vi "FTW-Endpoint-Connect.vi"(0 "FTW ØMQ Endpoint":refnum<class "FTW-Endpoint-ZMQ.lvclass">, 5 "Endpoint Address":T1, 11 "error in":errorcluster) -> (4 "FTW ØMQ Endpoint out":refnum<class "FTW-Endpoint-ZMQ.lvclass">, 15 "error out":errorcluster)   [LabVIEW 2012, in "FTW-Actor.lvlib" / "FTW-Endpoint-ZMQ.lvclass"]
uses:
  FTW-Endpoint-ZMQ.lvclass
  Utility/FTW-Actor-Address.ctl
  FTW-Endpoint-ZMQ.lvclass/FTW-Endpoint-ZMQ.ctl
  FTW-Actor.lvlib
panel:
  # "Inputs"
  # "Outputs"
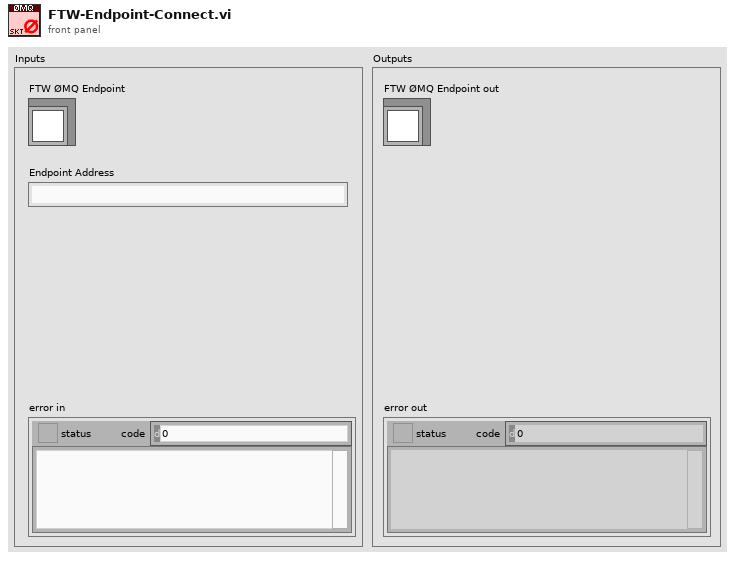
[diagram p1: front panel]
types:
  T1 = typedef "FTW-Actor.lvlib/FTW-Actor-Address.ctl" = string
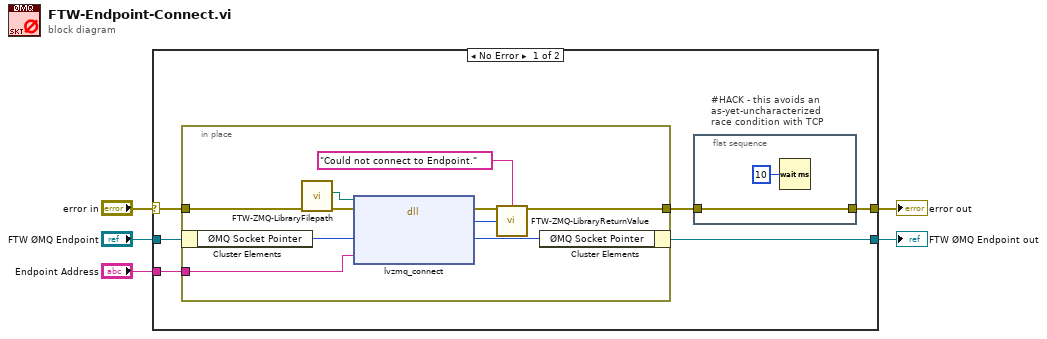
[diagram p0: block diagram]
diagram:
  n1 = case shown="No Error" "error in" {
    selector: "error in" -> [w9 w24]
    tunnel: "FTW ØMQ Endpoint" -> [w11 w25]
    tunnel: [w6 w24] -> w4
    tunnel: [w10 w25] -> w3
    tunnel: "Endpoint Address" -> [w8 _]
    frame No Error {
      n2 = in-place {
        in-place-border: w9 -> [w22]
        in-place-border: [w21] -> w7
        in-place-border: w8 -> [w20]
        n3 = in-place-cluster #1(w11) -> ("ØMQ Socket Pointer"=w23:u64)
        n4 = call "FTW-ZMQ-LibraryFilepath.vi"("error in"=w22) -> ("error out"=w15:errorcluster, "FTW-ZMQ Library Filepath"=w14:path)  [unwired: 8 in, 1 out]
        n5 = dll-call lib="?" fn="lvzmq_connect" ("zmq_labview.dll:lvzmq_bind")(path in=w14, error in=w15, "Socket Pointer"=w23, "Endpoint"=w20) -> (error out=w18:errorcluster, "Return Value"=w17:i32, "Socket Pointer"=w19:u64)  [unwired: 2 in, 1 out]
        n6 = call "FTW-ZMQ-LibraryReturnValue.vi"("error in"=w18, "Error Message"="Could not connect to Endpoint.", "Return Value"=w17) -> ("error out"=w21:errorcluster)  [unwired: 12 in]
        n7 = in-place-cluster #1("ØMQ Socket Pointer"=w19) -> (w10:refnum<class "FTW-Endpoint-ZMQ.lvclass">)
      }
      n8 = flat-sequence "#HACK - this avoids an\nas-yet-uncharacterized\nrace condition with TCP" {
        tunnel: [w13] -> w6
        tunnel: w7 -> [w13]
        frame #0 {
          n9 = Wait (ms)(milliseconds to wait=u32 10) -> ()  [unwired: 1 out]
        }
      }
    }
    frame Error {
    }
  }
  "error out" <- w4
  "FTW ØMQ Endpoint out" <- w3
